vi "Ball Shooter Global.vi"() -> ()   [LabVIEW 2016]
panel:
  in  "Shooter Wheel RPM":dbl
  in  "Intake Belt RPM":dbl
  in  "Grinder Power":dbl
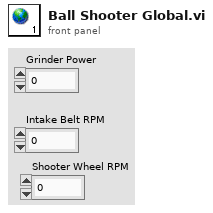
[diagram p1: front panel]
diagram:
